vi "Update_Global.vi"() -> ()   [LabVIEW 2010]
panel:
  in  "Location":string="/~FRC/EnFlo_Software_Site/Software/Enflo%20Software/"
  in  "Web site (URL)":string="midsummer.mech.surrey.ac.uk"
  in  "Source Folder":path
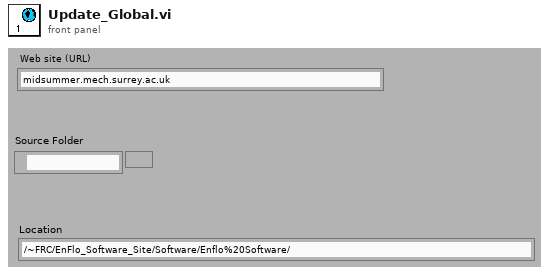
[diagram p1: front panel]
diagram:
